vi "JSON to LVObject - Invalid Type in nested Class - Returns Error.vi"() -> ()   [LabVIEW 2017, in "Generic Object Serializer Tests.lvlib"]
uses:
  Generic Object Serializer Tests.lvlib
  Generic Object Serializer/Generic Object Serializer.lvclass
  City/City.lvclass
  Generic Object Serializer/Type Name Handling.ctl
  Generic Object Serializer/Generic Object Serializer.lvclass/Generic Object Serializer.ctl
  Generic Object Serializer/Write Type Name Handling.vi
  <vilib>/addons/_JKI Toolkits/Caraya/classes/Assert/Assert Error.vi
  <vilib>/addons/_JKI Toolkits/Caraya/classes/Test/Test.lvclass
  <vilib>/addons/_JKI Toolkits/Caraya/classes/Assert/Assert.lvclass
panel:
  out "error out":errorcluster
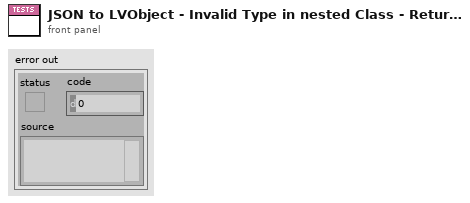
[diagram p1: front panel]
types:
  T1 = typedef "Generic Object Serializer.lvclass/Type Name Handling.ctl" = enum16{"None", "Inline"}
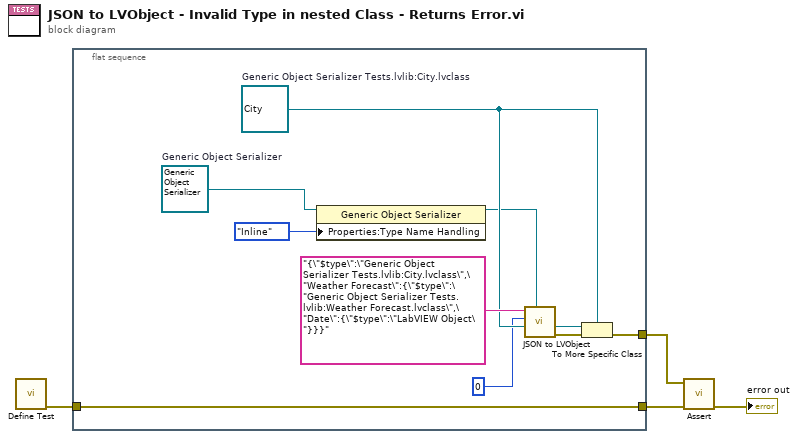
[diagram p0: block diagram]
diagram:
  n1 = call <vilib>:"Define Test.vi"() -> ("error out"=w4:errorcluster)  [unwired: 11 in]
  n2 = flat-sequence {
    tunnel: w4 -> [w9]
    tunnel: [w11] -> w2
    tunnel: [w9] -> w1
    frame #0 {
      w8 = refnum<class "City.lvclass"> refnum  # Generic Object Serializer Tests.lvlib:City.lvclass
      w14 = refnum<class "Generic Object Serializer.lvclass"> refnum  # Generic Object Serializer
      n3 = property class="Generic Object Serializer"(reference=w14, "Properties:Type Name Handling"=Type_Name_Handling."Inline" ("Type Name Handling")) -> (reference out=w6:refnum<class "Generic Object Serializer.lvclass">)  [unwired: 1 in, 1 out]
      n4 = call-dynamic "JSON to LVObject.vi"("LVClass Serializer"=w6, "Object Type"=w8, "Offset"=0, "JSON"="{\"$type\":\"Generic Object Serializer Tests.lvlib:City.lvclass\",\"Weather Forecast\":{\"$type\":\"Generic Object Serializer Tests.lvlib:Weather Forecast.lvclass\",\"Date\":{\"$type\":\"LabVIEW Object\"}}}") -> ("error out"=w13:errorcluster, "Object"=w10:refnum<class>)  [unwired: 6 in]
      n5 = To More Specific Class(target class=w8, reference=w10, error in=w13) -> (error out=w11:errorcluster)  [unwired: 1 out]
    }
  }
  n6 = call-poly <vilib>:"Assert.vi"("error in (no error)"=w1, "Error?"=w2) -> ("error out"=→"error out":errorcluster)  [unwired: 9 in]
